vi "OE2031&OE2041_Configure Ref Phase.vi"(7 "OE2041_Configure Ref Phase":T1={"Reference Source"=0, "Sweep Mode"=0, "Start Frequency(Hz)"=1000.0, "Stop Frequency(Hz)"=5000.0, "Linear Step Frequency(Hz)"=1000.0, "Log Step Percent(%)"=10.0, "Step Time(ms)"=1000, "Sweep Run Mode"=0, "Internal Frequency(Hz)"=1000.0, "Phase  (degree)"=0.0, "External Ref Trigger"=0, "Instrument Mode "=8} {"Instrument Mode" items=["OE2031-10M"=6, "OE2041-30M"=7, "OE2041-60M"=8]; "External Ref Trigger" items=["TTL Rising Edge", "Sine Zero Crossing"]; "Phase  (degree)" min=-180.0 max=180.0 format="%#.2g"; "Internal Frequency(Hz)" min=1e-05 max=60000000.0 format="%#.3f"; "Sweep Run Mode" items=["Stop", "Singal", "Loop"]; "Log Step Percent(%)" min=-100.0 max=100.0 format="%#.2f"; "Linear Step Frequency(Hz)" min=1e-05 max=60000000.0 format="%#.3f"; "Stop Frequency(Hz)" min=1e-05 max=60000000.0 format="%#.3f"; "Start Frequency(Hz)" min=1e-05 max=60000000.0 format="%#.3f"; "Sweep Mode" items=["Linear", "Log"]; "Reference Source" items=["External", "Internal", "Internal Sweep", "Self"]}, 8 "Error in (no error)":errorcluster caption="error out（no error）", 9 "Remote Mode":u16(ring) items=["USB"=0, "RS232"=1, "Ethernet"=3], 10 "Connection ID in":refnum<k5>, 11 "VISA resource name":refnum<visa-resource-name>) -> (0 "Error out":errorcluster caption="error out", 1 "Output String":string, 2 "Connection ID out":refnum<k5>, 3 "VISA resource  out":refnum<visa-resource-name>)   [LabVIEW 2011]
panel:
  out "字符串":string
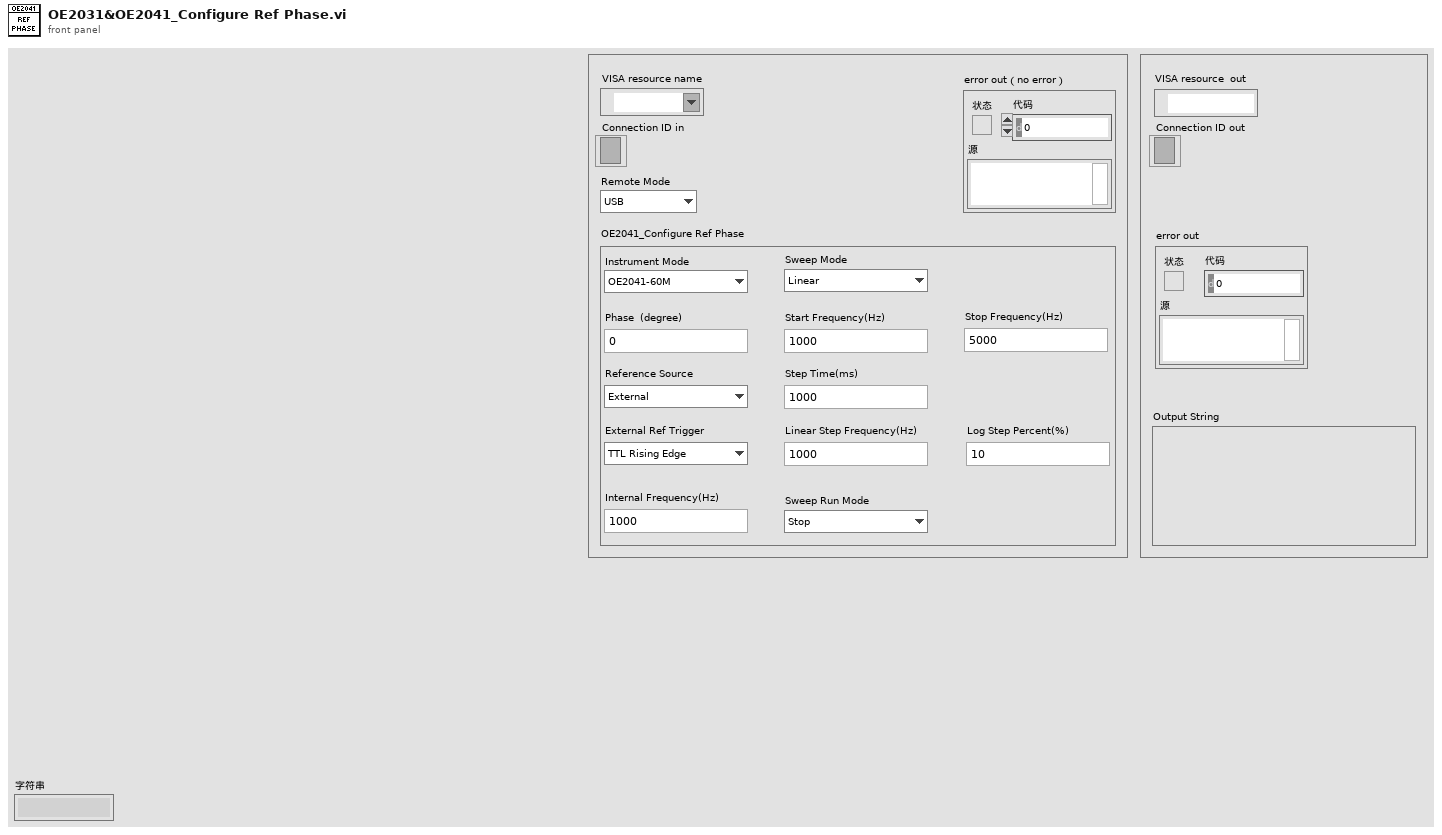
[diagram p1: front panel]
types:
  T1 = cluster{"Reference Source":u16, "Sweep Mode":u16, "Start Frequency(Hz)":dbl, "Stop Frequency(Hz)":dbl, "Linear Step Frequency(Hz)":dbl, "Log Step Percent(%)":dbl, "Step Time(ms)":i32, "Sweep Run Mode":u16, "Internal Frequency(Hz)":dbl, "Phase  (degree)":dbl, "External Ref Trigger":u16, "Instrument Mode ":u16}
  T2 = enum16{"ISRC", "IGND", "ICPL", "ILIN", "PHAS", "FMOD", "RSLP", "FREQ", "SWPT", "SLLM", "SULM", "SSLL", "SSLG", "STLM", "SWRM", "IRNG", "SENS", "RMOD", "OFLT", "OFSL", "SYNC", "DMOD", "HARM", "DARB", "SWVT", "SLVL", "SVLL", "SVUL", "SVSL", "SVSG", "SVTM", "SVRM", "RALL", "SNAP", "OUTP", "OAUX", "COUT", "CAUX", "COFP", "CEXP", "FPOP", "OEXP", "*IDN", "*RST", "OVLD", "INOV", "GNOV", "*PLL", "SSET", "RSET", "AGAN", "APHS", "ARSV", "ASCL", "EQCD", "EQCS", "SPED", "SRAT", "SLEN", "SSLE", "STRG", "SPRM", "STRD", "PAUS", "REST", "SPTS", "TRCA", "TEMP", "RSTU", "IHNZ", "DEQU", "SADD", "ARNG", "CSPE", "ISRCD", "IGNDD", "ICPLD", "ILIND", "PHASD", "FMODD", "RSLPD", "FREQD", "SWPTD", "SLLMD", "SULMD", "SSLLD", "SSLGD", "STLMD", "SWRMD", "SENSD", "RMODD", "OFLTD", "OFSLD", "SYNCD", "HARMD", "EQCDD", "EQCSD", "SNAPD", "OUTPD", "SWVTD", "SLVLD", "SVLLD", "SVULD", "SVSLD", "SVSGD", "SVTMD", "SVRMD", "SVDCD", "ARSVD", "AGAND", "APHSD", "ASCLD", "FPOPD", "CAUXD", "OEXPD", "SPEDD", "SRATD", "SLEND", "SSLED", "STRGD", "SPRMD", "STRDD", "PAUSD", "RESTD", "SPTSD", "TRCAD", "*IDND", "*RSTD", "INOVD", "GNOVD", "*PLLD", "SSETD", "RSETD", "RALLD"}
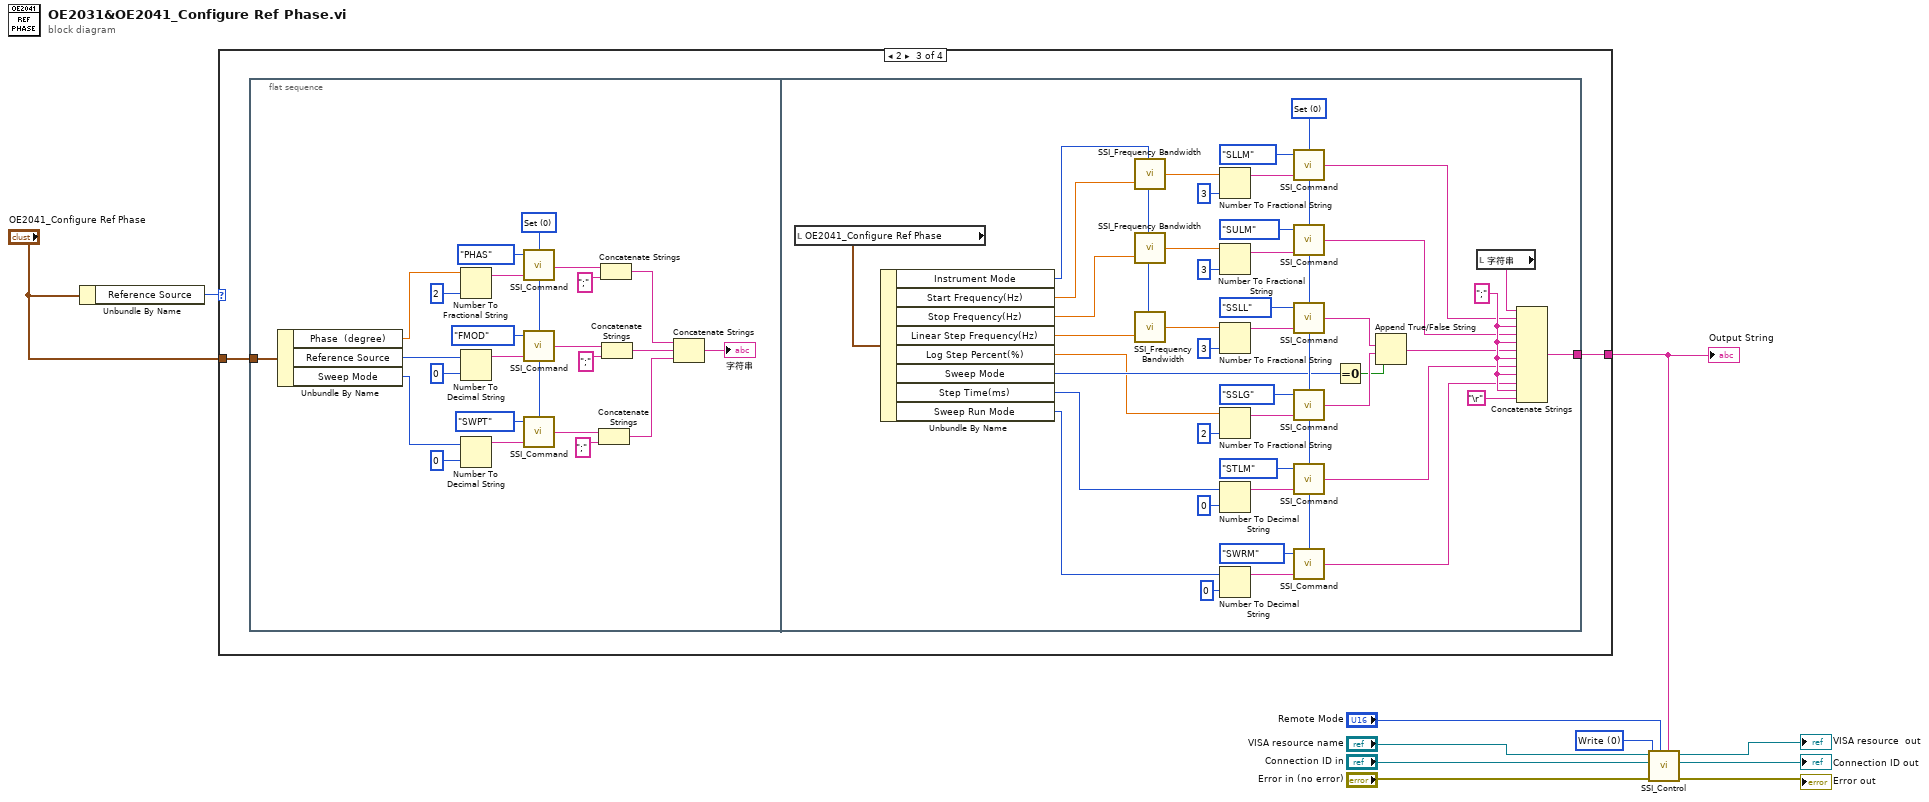
[diagram p0: block diagram]
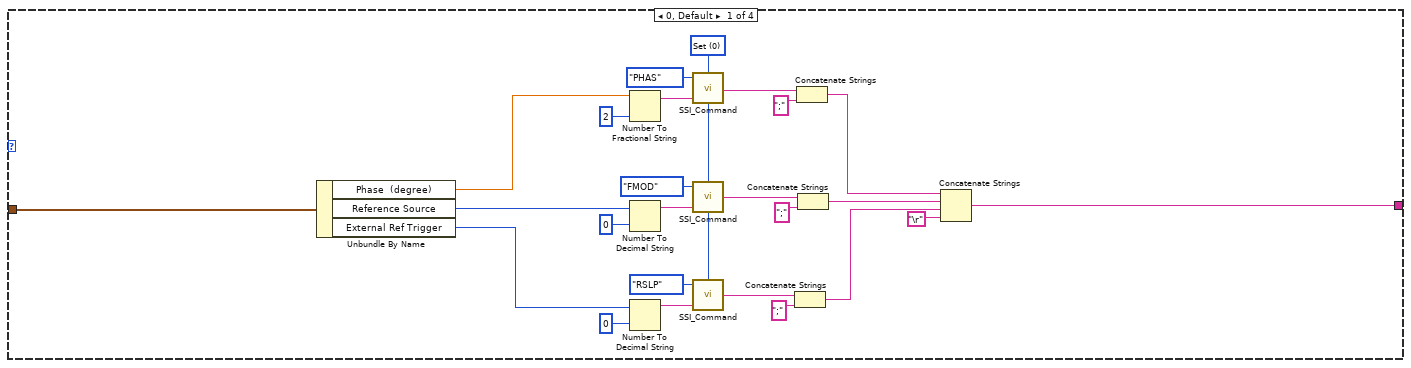
[diagram p2: hidden frame]
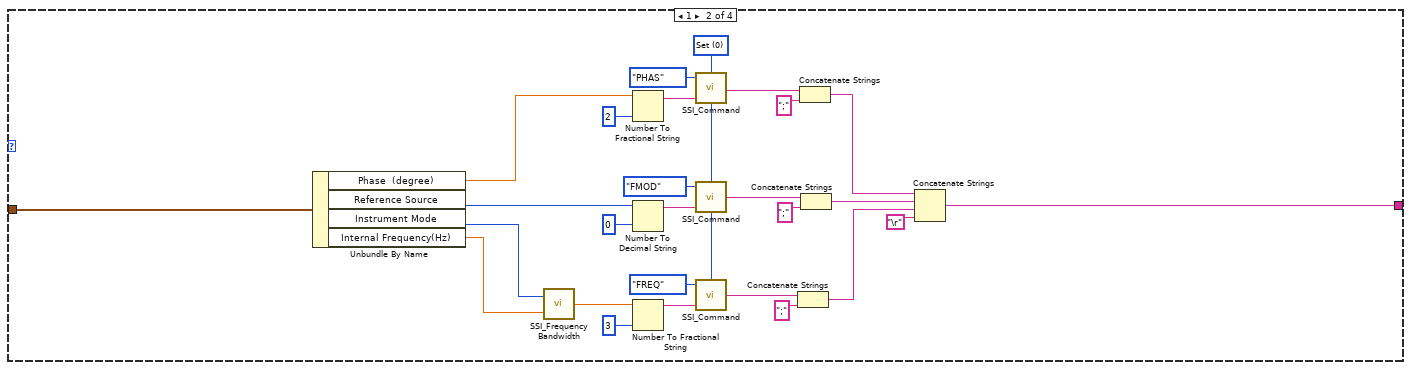
[diagram p3: hidden frame]
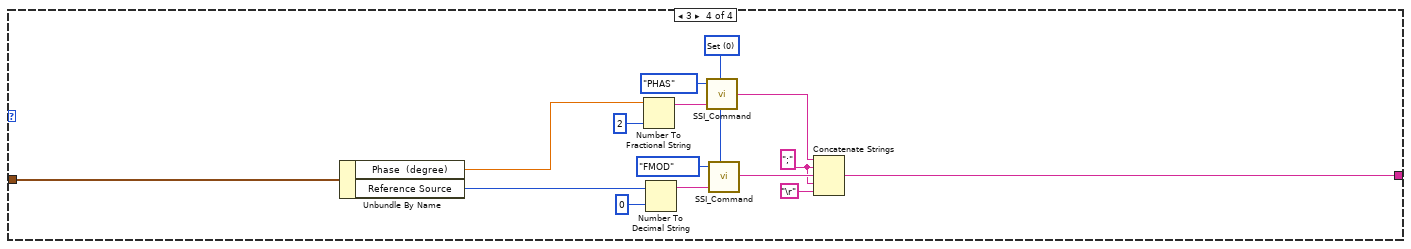
[diagram p4: hidden frame]
diagram:
  w9 = u16 0 items=["Write", "Read"] ("Control")
  n1 = Unbundle By Name("OE2041_Configure Ref Phase") -> ("Reference Source"=w2:u16)
  n2 = case shown="2" w2 {
    tunnel: "OE2041_Configure Ref Phase" -> [w23 w46 w65 w143]
    tunnel: [w17 w45 w64 w140] -> w3
    frame 0, Default {
      w22 = u16 0 items=["Set", "Query"] ("Opera")
      n3 = Unbundle By Name(w23) -> ("Phase  (degree)"=w12:dbl, "Reference Source"=w21:u16, "External Ref Trigger"=w24:u16)
      n4 = Number To Fractional String(number=w12, precision (6)=i16 2 ("精度(6)")) -> (F-format string=w35:string)  [unwired: 2 in]
      n5 = Number To Decimal String(number=w21, width (-)=i16 0 ("精度(6)")) -> (decimal integer string=w33:string)
      n6 = Number To Decimal String(number=w24, width (-)=i16 0 ("精度(6)")) -> (decimal integer string=w31:string)
      n7 = call "SSI_Command.vi"("Opera"=w22, "Paramter"=w35, "Command Type"=T2."PHAS") -> ("Output string"=w25:string)  [unwired: 1 in]
      n8 = call "SSI_Command.vi"("Opera"=w22, "Paramter"=w33, "Command Type"=T2."FMOD") -> ("Output string"=w27:string)  [unwired: 1 in]
      n9 = call "SSI_Command.vi"("Opera"=w22, "Paramter"=w31, "Command Type"=T2."RSLP") -> ("Output string"=w30:string)  [unwired: 1 in]
      n10 = Concatenate Strings(w30, ";" ("替换字符串(\"\")")) -> (w18:string)
      n11 = Concatenate Strings(w25, ";" ("替换字符串(\"\")")) -> (w20:string)
      n12 = Concatenate Strings(w27, ";" ("替换字符串(\"\")")) -> (w19:string)
      n13 = Concatenate Strings(w20, w19, w18, "\r") -> (w17:string)
    }
    frame 1 {
      w51 = u16 0 items=["Set", "Query"] ("Opera")
      n14 = Unbundle By Name(w46) -> ("Phase  (degree)"=w41:dbl, "Reference Source"=w50:u16, "Instrument Mode"=w37:u16, "Internal Frequency(Hz)"=w38:dbl)
      n15 = call "SSI_Frequency Bandwidth.vi"("Frequency"=w38, "Instrument Mode"=w37) -> ("Output"=w39:dbl)  [unwired: 1 in]
      n16 = Number To Fractional String(number=w41, precision (6)=i16 2 ("精度(6)")) -> (F-format string=w62:string)  [unwired: 2 in]
      n17 = Number To Decimal String(number=w50, width (-)=i16 0 ("精度(6)")) -> (decimal integer string=w60:string)
      n18 = Number To Fractional String(number=w39, precision (6)=i16 3 ("精度(6)")) -> (F-format string=w58:string)  [unwired: 2 in]
      n19 = call "SSI_Command.vi"("Opera"=w51, "Paramter"=w62, "Command Type"=T2."PHAS") -> ("Output string"=w52:string)  [unwired: 1 in]
      n20 = call "SSI_Command.vi"("Opera"=w51, "Paramter"=w60, "Command Type"=T2."FMOD") -> ("Output string"=w54:string)  [unwired: 1 in]
      n21 = call "SSI_Command.vi"("Opera"=w51, "Paramter"=w58, "Command Type"=T2."FREQ") -> ("Output string"=w57:string)  [unwired: 1 in]
      n22 = Concatenate Strings(w57, ";" ("替换字符串(\"\")")) -> (w47:string)
      n23 = Concatenate Strings(w52, ";" ("替换字符串(\"\")")) -> (w49:string)
      n24 = Concatenate Strings(w54, ";" ("替换字符串(\"\")")) -> (w48:string)
      n25 = Concatenate Strings(w49, w48, w47, "\r") -> (w45:string)
    }
    frame 2 {
      n26 = flat-sequence {
        tunnel: w65 -> [w71]
        tunnel: [w102] -> w64
        frame #0 {
          w76 = u16 0 items=["Set", "Query"] ("Opera")
          n27 = Unbundle By Name(w71) -> ("Phase  (degree)"=w69:dbl, "Reference Source"=w75:u16, "Sweep Mode"=w77:u16)
          n28 = Number To Fractional String(number=w69, precision (6)=i16 2 ("精度(6)")) -> (F-format string=w88:string)  [unwired: 2 in]
          n29 = Number To Decimal String(number=w75, width (-)=i16 0 ("精度(6)")) -> (decimal integer string=w86:string)
          n30 = Number To Decimal String(number=w77, width (-)=i16 0 ("精度(6)")) -> (decimal integer string=w84:string)
          n31 = call "SSI_Command.vi"("Opera"=w76, "Paramter"=w88, "Command Type"=T2."PHAS") -> ("Output string"=w78:string)  [unwired: 1 in]
          n32 = call "SSI_Command.vi"("Opera"=w76, "Paramter"=w86, "Command Type"=T2."FMOD") -> ("Output string"=w80:string)  [unwired: 1 in]
          n33 = call "SSI_Command.vi"("Opera"=w76, "Paramter"=w84, "Command Type"=T2."SWPT") -> ("Output string"=w83:string)  [unwired: 1 in]
          n34 = Concatenate Strings(w83, ";" ("替换字符串(\"\")")) -> (w72:string)
          n35 = Concatenate Strings(w78, ";" ("替换字符串(\"\")")) -> (w74:string)
          n36 = Concatenate Strings(w80, ";" ("替换字符串(\"\")")) -> (w73:string)
          n37 = Concatenate Strings(w74, w73, w72) -> (→"字符串":string)
        }
        frame #1 {
          w132 = ";"
          w122 = u16 0 items=["Set", "Query"] ("Opera")
          n38 = local read "OE2041_Configure Ref Phase"() -> (w98:T1)
          n39 = Unbundle By Name(w98) -> ("Instrument Mode"=w97:u16, "Start Frequency(Hz)"=w106:dbl, "Stop Frequency(Hz)"=w105:dbl, "Linear Step Frequency(Hz)"=w104:dbl, "Log Step Percent(%)"=w90:dbl, "Sweep Mode"=w101:u16, "Step Time(ms)"=w100:i32, "Sweep Run Mode"=w99:u16)
          n40 = call "SSI_Frequency Bandwidth.vi"("Frequency"=w106, "Instrument Mode"=w97) -> ("Output"=w109:dbl)  [unwired: 1 in]
          n41 = call "SSI_Frequency Bandwidth.vi"("Frequency"=w105, "Instrument Mode"=w97) -> ("Output"=w108:dbl)  [unwired: 1 in]
          n42 = call "SSI_Frequency Bandwidth.vi"("Frequency"=w104, "Instrument Mode"=w97) -> ("Output"=w107:dbl)  [unwired: 1 in]
          n43 = Number To Fractional String(number=w109, precision (6)=i16 3 ("精度(6)")) -> (F-format string=w118:string)  [unwired: 2 in]
          n44 = Number To Fractional String(number=w108, precision (6)=i16 3 ("精度(6)")) -> (F-format string=w116:string)  [unwired: 2 in]
          n45 = Number To Fractional String(number=w107, precision (6)=i16 3 ("精度(6)")) -> (F-format string=w114:string)  [unwired: 2 in]
          n46 = Number To Fractional String(number=w90, precision (6)=i16 2 ("精度(6)")) -> (F-format string=w112:string)  [unwired: 2 in]
          n47 = Number To Decimal String(number=w100, width (-)=i16 0 ("精度(6)")) -> (decimal integer string=w110:string)
          n48 = Number To Decimal String(number=w99, width (-)=i16 0 ("精度(6)")) -> (decimal integer string=w120:string)
          n49 = call "SSI_Command.vi"("Opera"=w122, "Paramter"=w118, "Command Type"=T2."SLLM") -> ("Output string"=w126:string)  [unwired: 1 in]
          n50 = call "SSI_Command.vi"("Opera"=w122, "Paramter"=w116, "Command Type"=T2."SULM") -> ("Output string"=w127:string)  [unwired: 1 in]
          n51 = call "SSI_Command.vi"("Opera"=w122, "Paramter"=w114, "Command Type"=T2."SSLL") -> ("Output string"=w124:string)  [unwired: 1 in]
          n52 = call "SSI_Command.vi"("Opera"=w122, "Paramter"=w112, "Command Type"=T2."SSLG") -> ("Output string"=w125:string)  [unwired: 1 in]
          n53 = call "SSI_Command.vi"("Opera"=w122, "Paramter"=w110, "Command Type"=T2."STLM") -> ("Output string"=w129:string)  [unwired: 1 in]
          n54 = call "SSI_Command.vi"("Opera"=w122, "Paramter"=w120, "Command Type"=T2."SWRM") -> ("Output string"=w130:string)  [unwired: 1 in]
          n55 = Equal To 0?(x=w101) -> (x = 0?=w123:bool)
          n56 = Append True/False String(1:w123, 2:w125, 3:w124) -> (0:w128:string)  [unwired: 1 in]
          n57 = local read "字符串"() -> (w103:string)
          n58 = Concatenate Strings(w103, w126, w132, w127, w132, w128, w132, w129, w132, w130, w132, "\r") -> (w102:string)
        }
      }
    }
    frame 3 {
      w133 = u16 0 items=["Set", "Query"] ("Opera")
      w135 = ";" ("替换字符串(\"\")")
      n59 = Unbundle By Name(w143) -> ("Phase  (degree)"=w134:dbl, "Reference Source"=w144:u16)
      n60 = Number To Fractional String(number=w134, precision (6)=i16 2 ("精度(6)")) -> (F-format string=w138:string)  [unwired: 2 in]
      n61 = Number To Decimal String(number=w144, width (-)=i16 0 ("精度(6)")) -> (decimal integer string=w146:string)
      n62 = call "SSI_Command.vi"("Opera"=w133, "Paramter"=w138, "Command Type"=T2."PHAS") -> ("Output string"=w136:string)  [unwired: 1 in]
      n63 = call "SSI_Command.vi"("Opera"=w133, "Paramter"=w146, "Command Type"=T2."FMOD") -> ("Output string"=w145:string)  [unwired: 1 in]
      n64 = Concatenate Strings(w136, w135, w145, w135, "\r") -> (w140:string)
    }
  }
  "Output String" <- w3
  n65 = call "SSI_Control.vi"("Write Buffer"=w3, "Remote Mode"="Remote Mode", "Error in (no error)"="Error in (no error)", "Control"=w9, "Connection ID in"="Connection ID in", "VISA resource name"="VISA resource name") -> ("Error out"=→"Error out":errorcluster, "Connection ID out"=→"Connection ID out":refnum<k5>, "VISA resource  out"=→"VISA resource  out":refnum<visa-resource-name>)  [unwired: 2 in, 1 out]
